vi "PAQ_Table_read_all_samples.vi"(5 "Time-End":timestamp, 7 "Time-Start":timestamp, 8 "error in (no error)":errorcluster, 9 "Sub Path":path, 11 "Table Filename":string) -> (0 "error out":errorcluster, 1 "TAGs":string[](array[string]), 2 "Fetched samples":i32, 3 "Fetched PAQ-samples":T1)   [LabVIEW 2020, in "Sgraph_lib_V1.lvlib" / "DBAL-BIN.lvclass"]
doc: "Read all samples from one PAQ file"
uses:
  DBAL-BIN.lvclass
  controls/BIN/BINdata.ctl
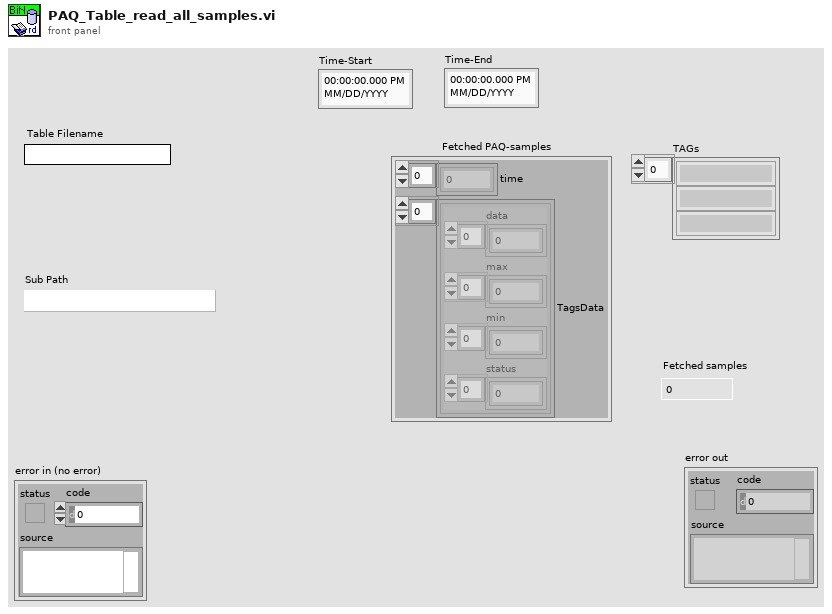
[diagram p1: front panel]
types:
  T1 = typedef "Sgraph_lib_V1.lvlib/DBAL-BIN.lvclass/BINdata.ctl" = cluster{"time":dbl[], "TagsData":cluster{"data":dbl[], "max":dbl[], "min":dbl[], "status":u32[]}[]}
  T2 = cluster{"data":dbl[], "max":dbl[], "min":dbl[], "status":u32[]}[]
  T3 = cluster{"data":dbl[], "max":dbl[], "min":dbl[], "status":u32[]}
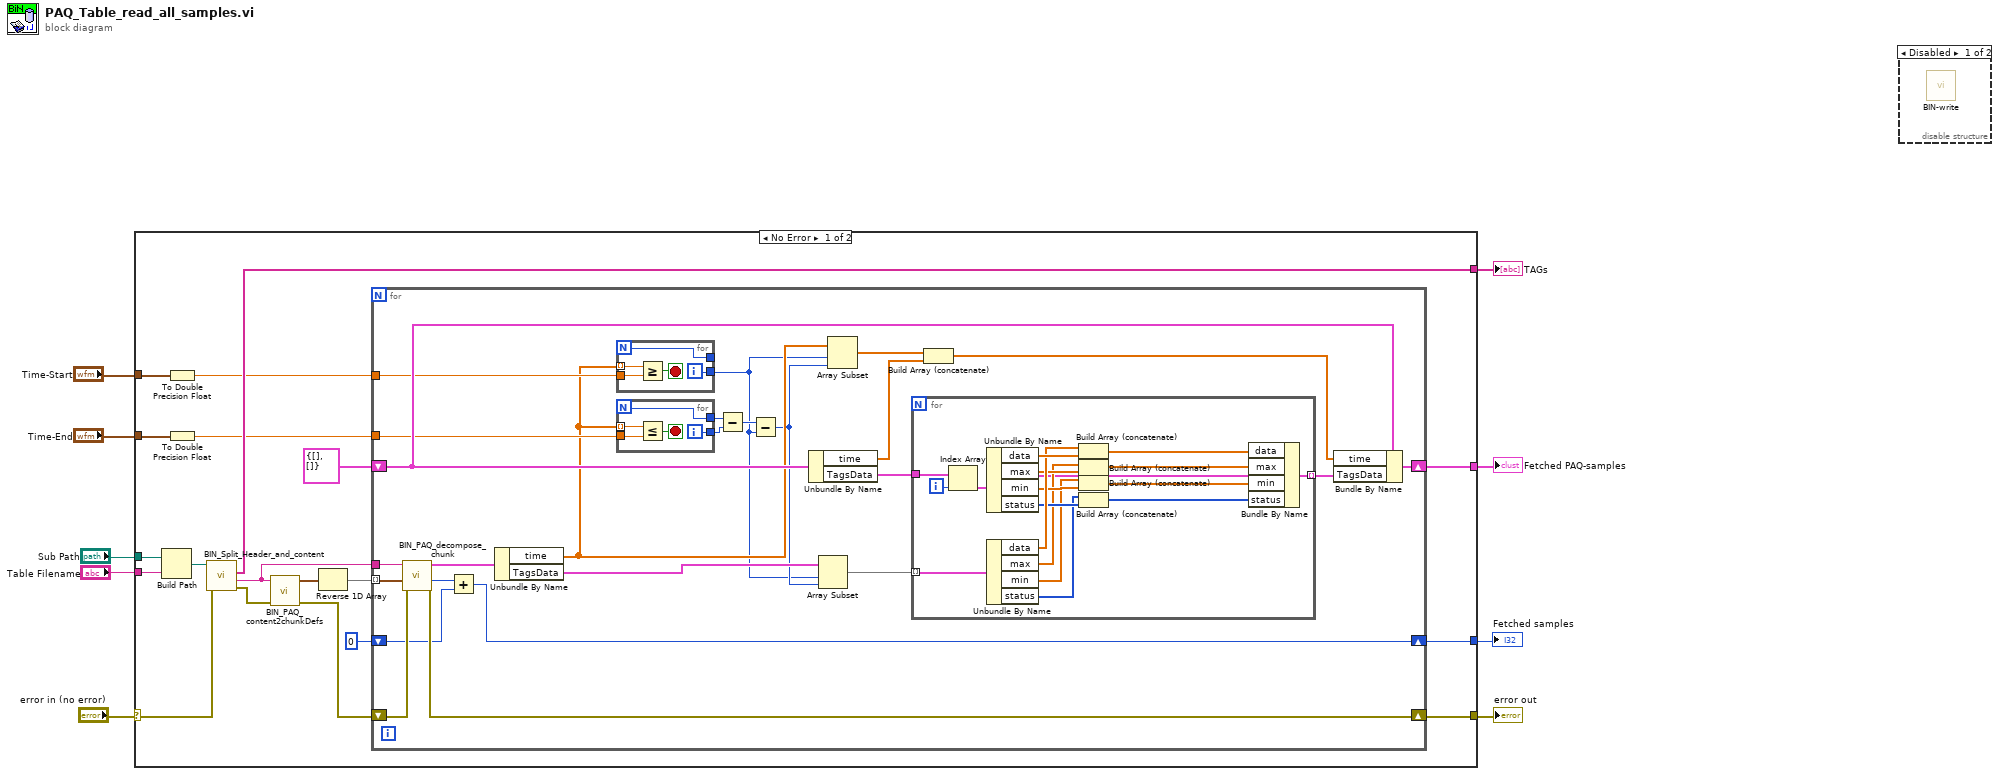
[diagram p0: block diagram]
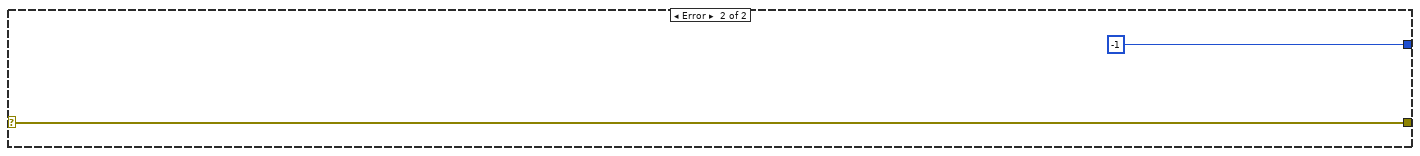
[diagram p3: hidden frame]
diagram:
  n1 = case shown="No Error" "error in (no error)" {
    selector: "error in (no error)" -> [w27 w82]
    tunnel: [w23 w82] -> w8
    tunnel: "Sub Path" -> [w15 _]
    tunnel: "Table Filename" -> [w14 _]
    tunnel: [w18 -1 ("Samples size")] -> w3
    tunnel: [w17 _] -> w5
    tunnel: [w16 _] -> w4
    tunnel: "Time-Start" -> [w13 _]
    tunnel: "Time-End" -> [w12 _]
    frame No Error {
      n2 = Build Path(base path=w15, name or relative path=w14) -> (appended path=w28:path)
      n3 = To Double Precision Float(number=w13) -> (double precision float=w10:dbl)
      n4 = To Double Precision Float(number=w12) -> (double precision float=w11:dbl)
      n5 = call "BIN_Split_Header_and_content.vi"("error in"=w27, "Path in"=w28) -> ("error out"=w26:errorcluster, "Content"=w25:string, "TAGs"=w16:string[])  [unwired: 5 in, 2 out]
      n6 = call "BIN_PAQ_content2chunkDefs.vi"("error in (no error)"=w26, "Content"=w25) -> ("error out"=w24:errorcluster, "Data segments"=w22:cluster{"Offset":u32, "Size":u32}[])  [unwired: 8 in]
      n7 = Reverse 1D Array(array=w22) -> (reversed array=w21:cluster{"Offset":u32, "Size":u32}[])
      n8 = for {
        tunnel: w21 -> [w53] mode=indexing
        tunnel: w25 -> [w52]
        shift-right: [w50] -> w23
        shift-left: w24 -> [w51]
        shift-right: [w41] -> w18
        shift-left: 0 ("Samples size") -> [w43]
        shift-right: [w48] -> w17
        shift-left: T1 {"time"=[], "TagsData"=[]} ("PAQ_data") -> [w49]
        tunnel: w11 -> [w40]
        tunnel: w10 -> [w37]
        n9 = call "BIN_PAQ_decompose_chunk.vi"("error in (no error)"=w51, "Offset"=w53, "Content"=w52) -> ("error out"=w50:errorcluster, "Samples size"=w44:i32, "PAQ_data"=w35:T1)  [unwired: 6 in]
        n10 = Add(x=w44, y=w43) -> (x+y=w41:i32)
        n11 = Unbundle By Name(w35) -> ("time"=w34:dbl[], "TagsData"=w32:T2)
        n12 = for {
          N -> [w55]
          tunnel: w34 -> [w58] mode=indexing
          tunnel: w37 -> [w57]
          tunnel: [w55] -> _
          tunnel: [w54] -> w29
          i -> [w54]
          stop <- w56 stop-if-true
          n13 = Greater Or Equal?(x=w58, y=w57) -> (x >= y?=w56:bool)
        }
        n14 = for {
          N -> [w60]
          tunnel: w34 -> [w63] mode=indexing
          tunnel: w40 -> [w62]
          tunnel: [w60] -> w39
          tunnel: [w59] -> w38
          i -> [w59]
          stop <- w61 stop-if-true
          n15 = Less Or Equal?(x=w63, y=w62) -> (x <= y?=w61:bool)
        }
        n16 = Subtract(x=w39, y=w38) -> (x-y=w36:i32)
        n17 = Subtract(x=w36, y=w29) -> (x-y=w31:i32)
        n18 = Unbundle By Name(w49) -> ("time"=w47:dbl[], "TagsData"=w46:T2)
        n19 = Array Subset(array=w32, index=w29, length=w31) -> (w30:T2)
        n20 = Array Subset(array=w34, index=w29, length=w31) -> (w33:dbl[])
        n21 = for {
          tunnel: w30 -> [w78] mode=indexing
          tunnel: w46 -> [w80]
          tunnel: [w68] -> w45 mode=indexing
          i -> [w79]
          n22 = Index Array(array=w80, index=w79) -> (element=w69:T3)
          n23 = Unbundle By Name(w69) -> ("data"=w77:dbl[], "max"=w75:dbl[], "min"=w74:dbl[], "status"=w73:u32[])
          n24 = Unbundle By Name(w78) -> ("data"=w76:dbl[], "max"=w70:dbl[], "min"=w71:dbl[], "status"=w72:u32[])
          n25 = Build Array (concatenate)(w76, w77) -> (w65:dbl[])
          n26 = Build Array (concatenate)(w70, w75) -> (w66:dbl[])
          n27 = Build Array (concatenate)(w71, w74) -> (w67:dbl[])
          n28 = Build Array (concatenate)(w72, w73) -> (w64:u32[])
          n29 = Bundle By Name(cluster=w69, "data"=w65, "max"=w66, "min"=w67, "status"=w64) -> (w68:T3)
        }
        n30 = Build Array (concatenate)(w33, w47) -> (w42:dbl[])
        n31 = Bundle By Name(cluster=w49, "time"=w42, "TagsData"=w45) -> (w48:T1)
      }
    }
    frame Error {
    }
  }
  "error out" <- w8
  "Fetched samples" <- w3
  "TAGs" <- w4
  "Fetched PAQ-samples" <- w5
  n32 = disable-structure shown="Disabled" {
    frame Disabled {
      n33 = call "BIN-write.vi"() -> ()  [unwired: 9 in, 3 out]
    }
    frame Enabled {
    }
  }
